vi "PFG600 update value.vi"(2 "Value":i16, 3 "Command":string) -> (0 "Text":string, 1 "Hex":string)   [LabVIEW 2023]
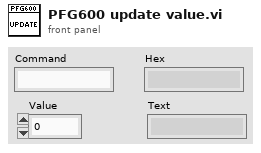
[diagram p1: front panel]
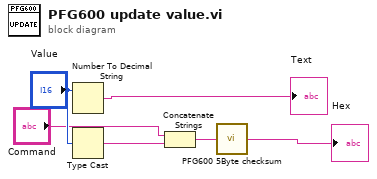
[diagram p0: block diagram]
diagram:
  n1 = Number To Decimal String(number="Value") -> (decimal integer string=→"Text":string)  [unwired: 1 in]
  n2 = Type Cast(x="Value") -> (*(type *) &x=w4:string)  [unwired: 1 in]
  n3 = Concatenate Strings("Command", w4) -> (w1:string)
  n4 = call "PFG600 5Byte checksum.vi"("Input"=w1) -> ("Output"=→"Hex":string)
